vi "read nodes.vi"() -> ()   [LabVIEW 2017, in "Lock-in module.lvlib"]
uses:
  <instrlib>/Zurich Instruments LabOne/Public/ziTypeHandle.ctl
  Lock-in module.lvlib
  <instrlib>/Zurich Instruments LabOne/Zurich Instruments LabOne.lvlib
panel:
  out "Nodes 2":string[][](array[string])=[["/FREQ", "", "", "", "", "", "", "", "", "", "", "", "", "", "", "", "", "", "", "", "", "", ""], ["/ADCSELECT", "/ORDER", "/RATE", "/OSCSELECT", "/HARMONIC", "/PHASESHIFT", "/SINC", "/BYPASS", "/TIMECONSTANT", "/ENABLE", "/FREQ", "/TRIGGER", "/PHASEADJUST", "/SAMPLE", "", "", "", "", "", "", "", "", ""], ["/ENABLE", "/AUTOMODE", "/ADCSELECT", "/DEMODSELECT", "/OSCSELECT", "/LOCKED", "", "", "", "", "", "", "", "", "", "", "", "", "", "", "", "", ""], ["", "", "", "", "", "", "", "", "", "", "", "", "", "", "", "", "", "", "", "", "", "", ""], ["", "", "", "", "", "", "", "", "", "", "", "", "", "", "", "", "", "", "", "", "", "", ""], ["", "", "", "", "", "", "", "", "", "", "", "", "", "", "", "", "", "", "", "", "", "", ""], ["/SAMPLE", "/AVERAGING", "/VALUES", "", "", "", "", "", "", "", "", "", "", "", "", "", "", "", "", "", "", "", ""], ["/WAVE", "/ENABLE", "/TIME", "/TRIGENABLE", "/TRIGRISING", "/TRIGFALLING", "/TRIGLEVEL", "/LENGTH", "/TRIGHOLDOFF", "/TRIGHOLDOFFCOUNT", "/TRIGHOLDOFFMODE", "/TRIGCHANNEL", "/CHANNELS", "/CHANNEL", "/SINGLE", "/TRIGHYSTERESIS", "/TRIGFORCE", "/TRIGSTATE", "/TRIGSLOPE", "/TRIGGATE", "/SEGMENTS", "/TRIGREFERENCE", "/TRIGDELAY"], ["/INPUT", "/EXTCLK", "/DECIMATION", "/MODE", "/DRIVE", "/OUTPUT", "/AUXDRIVE", "", "", "", "", "", "", "", "", "", "", "", "", "", "", "", ""], ["/DIFF", "/AC", "/IMP50", "/FLOAT", "/ON", "/RANGE", "/MIN", "/MAX", "/AUTORANGE", "/SCALING", "/RANGESTEP", "", "", "", "", "", "", "", "", "", "", "", ""], ["/RANGE", "/FLOAT", "/ON", "/MIN", "/MAX", "/AUTORANGE", "/SCALING", "/RANGESTEP", "", "", "", "", "", "", "", "", "", "", "", "", "", "", ""], ["/IMP50", "/DIFF", "/ON", "/RANGE", "/OVER", "/OFFSET", "/ADD", "/ENABLES", "/AMPLITUDES", "/AUTORANGE", "", "", "", "", "", "", "", "", "", "", "", "", ""], ["", "", "", "", "", "", "", "", "", "", "", "", "", "", "", "", "", "", "", "", "", "", ""], ["", "", "", "", "", "", "", "", "", "", "", "", "", "", "", "", "", "", "", "", "", "", ""], ["/VALUE", "/LIMITLOWER", "/LIMITUPPER", "/OUTPUTSELECT", "/DEMODSELECT", "/PREOFFSET", "/SCALE", "/OFFSET", "", "", "", "", "", "", "", "", "", "", "", "", "", "", ""], ["", "", "", "", "", "", "", "", "", "", "", "", "", "", "", "", "", "", "", "", "", "", ""], ["", "", "", "", "", "", "", "", "", "", "", "", "", "", "", "", "", "", "", "", "", "", ""]]
  out "Nodes":string[](array[string])=["OSCS", "DEMODS", "EXTREFS", "TRIGGERS", "STATUS", "STATS", "AUXINS", "SCOPES", "DIOS", "SIGINS", "CURRINS", "SIGOUTS", "SYSTEM", "FEATURES", "AUXOUTS", "TU", "CLOCKBASE"]
  out "Message":string="The API reports version18.12(revision: 59443 ), whilst the Data Server has version 18.12 (revision 59443 )"
  out "HandleOut":T1={"handleValid"=TRUE, "Conn"=347599416, "Path Prefix"="/DEV4029/", "Handle"=501862432, "Connected"=TRUE, "Clockbase(s)"=1.6666666666666667e-08} {"Handle" format="0x%08x"; "Conn" format="0x%08x"}
  out "Handle Out":T1={"handleValid"=FALSE, "Conn"=0, "Path Prefix"="/DEV4029/", "Handle"=0, "Connected"=FALSE, "Clockbase(s)"=1.6666666666666667e-08} {"Handle" format="0x%08x"; "Conn" format="0x%08x"}
  out "Selected Device":string="DEV4029"
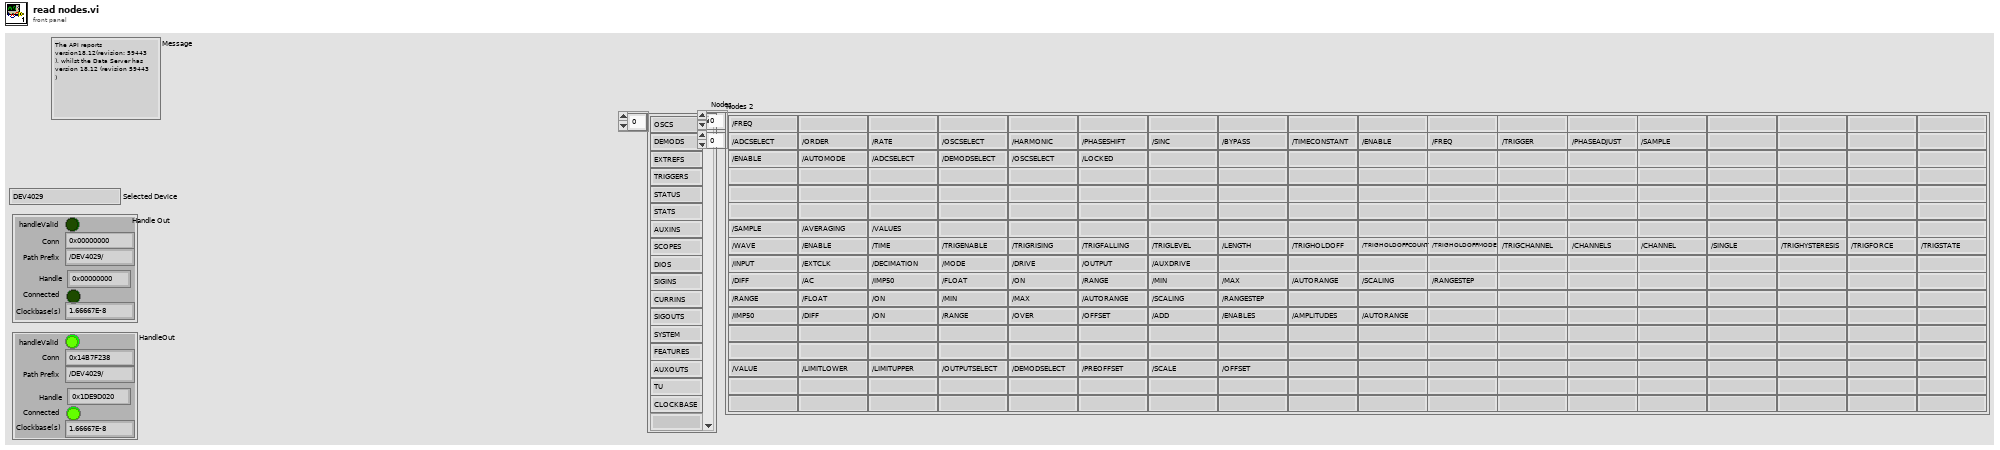
[diagram p1: front panel]
types:
  T1 = typedef "Zurich Instruments LabOne.lvlib/ziTypeHandle.ctl" = cluster{"handleValid":bool, "Conn":u64, "Path Prefix":string, "Handle":u64, "Connected":bool, "Clockbase(s)":dbl}
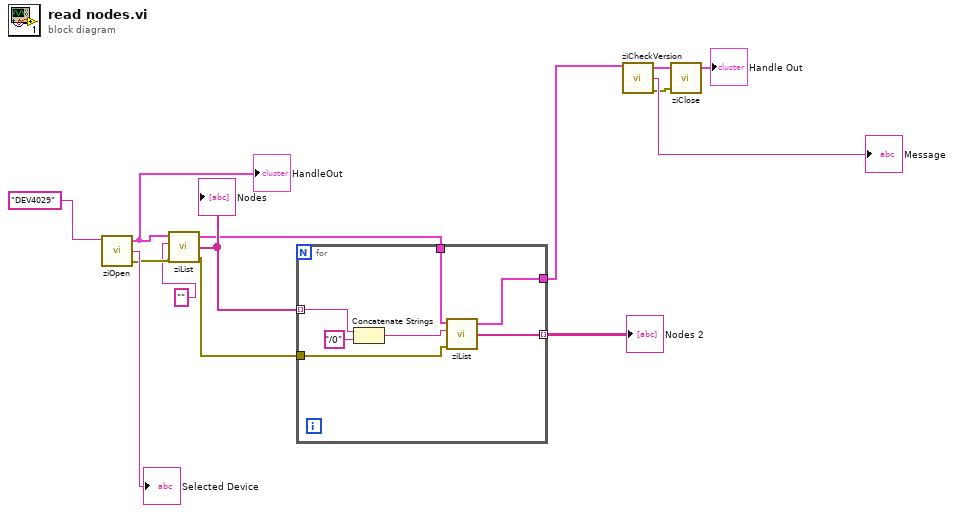
[diagram p0: block diagram]
diagram:
  n1 = call <instrlib>:"ziOpen.vi"("Address"="DEV4029") -> ("Error Out"=w7:errorcluster, "Selected Device"=→"Selected Device":string, "HandleOut"=w11:T1)  [unwired: 3 in]
  "HandleOut" <- w11
  n2 = call <instrlib>:"ziList.vi"("Error In"=w7, "Path (\"\")"="" ("Path (\"\")"), "Handle In"=w11) -> ("Error Out"=w3:errorcluster, "Nodes"=w5:string[], "Handle Out"=w4:T1)  [unwired: 1 in]
  "Nodes" <- w5
  n3 = for {
    tunnel: w5 -> [w20] mode=indexing
    tunnel: w4 -> [w19]
    tunnel: w3 -> [w17]
    tunnel: [w16] -> w2
    tunnel: [w15] -> w1 mode=indexing
    n4 = Concatenate Strings(w20, "/0" ("string")) -> (w18:string)
    n5 = call <instrlib>:"ziList.vi"("Error In"=w17, "Path (\"\")"=w18, "Handle In"=w19) -> ("Nodes"=w15:string[], "Handle Out"=w16:T1)  [unwired: 1 in, 1 out]
  }
  "Nodes 2" <- w1
  n6 = call <instrlib>:"ziCheckVersion.vi"("Handle In"=w2) -> ("Handle Out"=w9:T1, "Message"=→"Message":string, "Error Out"=w8:errorcluster)  [unwired: 12 in]
  n7 = call <instrlib>:"ziClose.vi"("Error In"=w8, "Handle In"=w9) -> ("Handle Out"=→"Handle Out":T1)  [unwired: 2 in, 1 out]
